vi "Call Function.vi"(8 "error in":errorcluster, 9 "Arguments":string, 10 "Function Name":string, 11 "Spark Reference In":T1) -> (0 "error out":errorcluster, 2 "Function Response":T4, 3 "Spark Reference Out":T1)   [LabVIEW 2013, in "Spark API.lvlib"]
uses:
  Controls/Spark Reference.ctl
  <vilib>/httpClient/ClientHandle.ctl
  Controls/Device Query JSON.ctl
  Controls/Function Response JSON.ctl
  Controls/Query Error JSON.ctl
  <vilib>/httpClient/POSTBuffer.vi
  Spark API.lvlib
  <vilib>/httpClient/LabVIEWHTTPClient.lvlib
panel:
  out "body":string
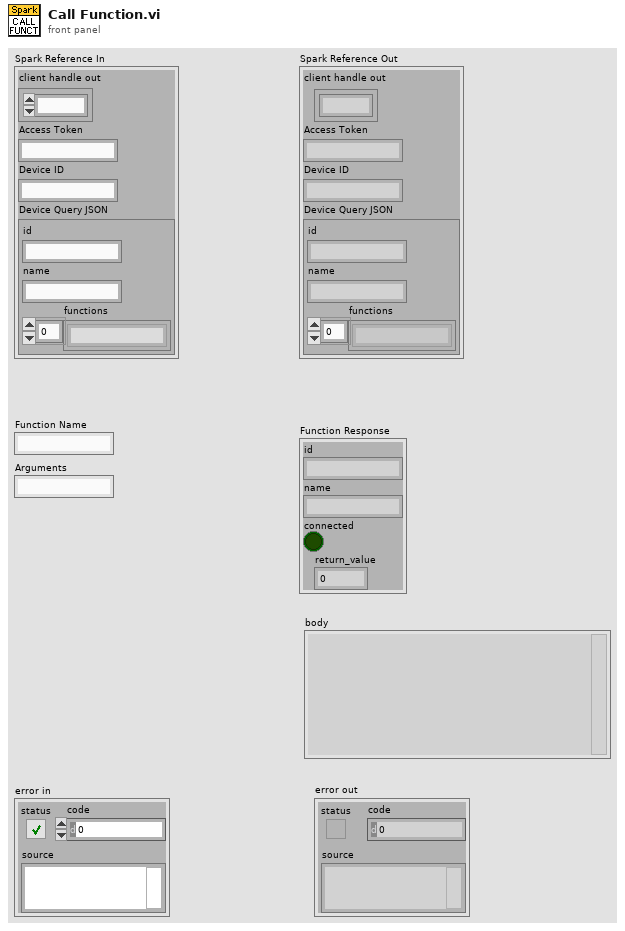
[diagram p1: front panel]
types:
  T1 = typedef "Spark API.lvlib/Spark Reference.ctl" = cluster{"client handle out":T2, "Access Token":string, "Device ID":string, "Device Query JSON":T3}
  T2 = typedef "LabVIEWHTTPClient.lvlib/ClientHandle.ctl" = refnum<k1>
  T3 = typedef "Spark API.lvlib/Device Query JSON.ctl" = cluster{"id":string, "name":string, "functions":string[]}
  T4 = cluster{"id":string, "name":string, "connected":bool, "return_value":dbl}
  T5 = typedef "Spark API.lvlib/Function Response JSON.ctl" = cluster{"id":string, "name":string, "connected":bool, "return_value":dbl}
  T6 = typedef "Spark API.lvlib/Query Error JSON.ctl" = cluster{"code":dbl, "error":string, "error description":string}
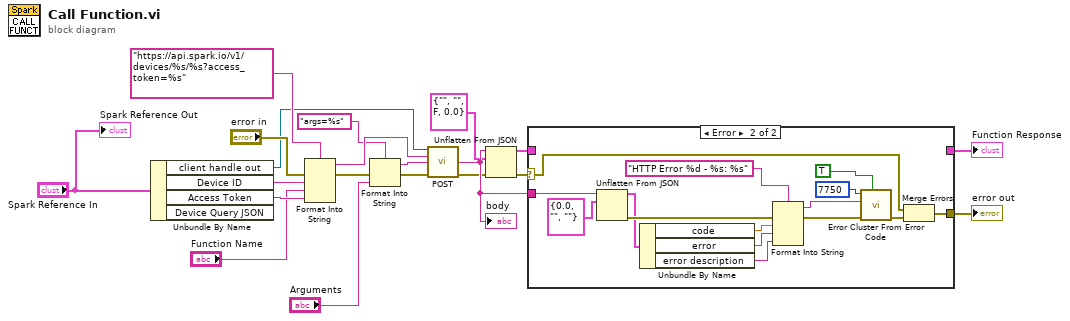
[diagram p0: block diagram]
diagram:
  n1 = Unbundle By Name("Spark Reference In") -> ("client handle out"=w15:T2, "Device ID"=w14:string, "Access Token"=w13:string)  [unwired: 1 out]
  n2 = Format Into String(format string="https://api.spark.io/v1/devices/%s/%s?access_token=%s" ("url"), error in="error in", w14, "Function Name", w13) -> (resulting string=w19:string, error out=w2:errorcluster)  [unwired: 1 in]
  n3 = Format Into String(format string="args=%s", error in=w2, "Arguments") -> (resulting string=w9:string, error out=w1:errorcluster)  [unwired: 1 in]
  n4 = call-poly <vilib>:"POST.vi"("client handle"=w15, "url"=w19, "buffer"=w9, "error in (no error)"=w1) -> ("body"=w7:string, "error out"=w6:errorcluster)  [unwired: 8 in, 2 out]
  "body" <- w7
  n5 = Unflatten From JSON(JSON string=w7, type and defaults=T5 {"id"="", "name"="", "connected"=FALSE, "return_value"=0.0} ("Function Response"), error in (no error)=w6) -> (value=w5:T5, error out=w3:errorcluster)  [unwired: 4 in]
  n6 = case shown="Error" w3 {
    selector: w3 -> [w21 w36]
    tunnel: w5 -> [w22 _]
    tunnel: [w21 w35] -> w17
    tunnel: w7 -> [_ w37]
    tunnel: [w22 _] -> w8
    frame No Error {
    }
    frame Error {
      n7 = Unflatten From JSON(JSON string=w37, type and defaults=T6 {"code"=0.0, "error"="", "error description"=""} ("Error JSON")) -> (value=w23:T6, error out=w26:errorcluster)  [unwired: 5 in]
      n8 = Unbundle By Name(w23) -> ("code"=w31:dbl, "error"=w30:string, "error description"=w29:string)
      n9 = Format Into String(format string="HTTP Error %d - %s: %s", error in=w26, w31, w30, w29) -> (resulting string=w28:string, error out=w27:errorcluster)  [unwired: 1 in]
      n10 = call <vilib>:"Error Cluster From Error Code.vi"("show call chain? (False)"=TRUE, "error in (no error)"=w27, "error message (\"\")"=w28, "error code (0)"=7750) -> ("error out"=w25:errorcluster)  [unwired: 5 in]
      n11 = Merge Errors(w36, w25) -> (w35:errorcluster)
    }
  }
  "error out" <- w17
  "Function Response" <- w8
  "Spark Reference Out" <- "Spark Reference In"
